vi "Cancel Download.vi"(8 "Error In":errorcluster, 11 "Download":T1) -> (0 "Error Out":errorcluster, 3 "Download":T1)   [LabVIEW 2020, in "LMH-Toolbox.lvlib"]
doc: "Cancel Download."
uses:
  LMH-Toolbox.lvlib
  Private/Web/Type Defs/Download Task.ctl
  Private/Web/LMH-Web.lvlib
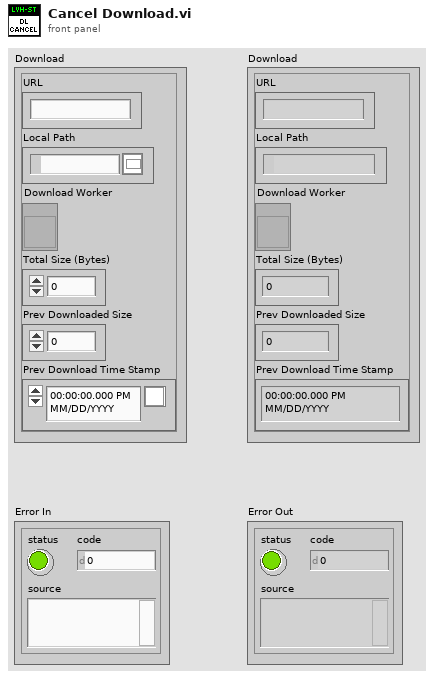
[diagram p1: front panel]
types:
  T1 = typedef "LMH-Toolbox.lvlib/LMH-Web.lvlib/Download Task.ctl" = cluster{"URL":string, "Local Path":path, "Download Worker":refnum<vi>, "Total Size (Bytes)":u64, "Prev Downloaded Size":u64, "Prev Download Time Stamp":timestamp}
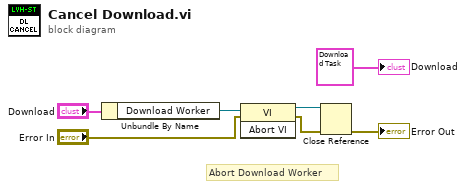
[diagram p0: block diagram]
diagram:
  # "Abort Download Worker"
  n1 = Unbundle By Name("Download") -> ("Download Worker"=w5:refnum<vi>)
  n2 = invoke class="VI" method="Abort VI"(reference=w5, error in="Error In") -> (reference out=w7:refnum<vi>, error out=w6:errorcluster)  [unwired: 1 in, 1 out]
  n3 = Close Reference(reference=w7, error in (no error)=w6) -> (error out=→"Error Out":errorcluster)
  "Download" <- T1 {"URL"="", "Local Path"=path "", "Download Worker"=refnum, "Total Size (Bytes)"=0, "Prev Downloaded Size"=0, "Prev Download Time Stamp"=timestamp(0 s since 1904-01-01)} ("Download")
